vi "Format JSON.vi"(8 "error in (no error)":errorcluster, 11 "String":string) -> (0 "error out":errorcluster, 3 "String out":string)   [LabVIEW 2015, in "Project.lvclass"]
uses:
  Project.lvclass
panel:
  # "Test:5"
  # "\"Test:5,Test1:6\""
  # "\"{\"\"Test\"\":5,\"\"Test1\"\":6}\""
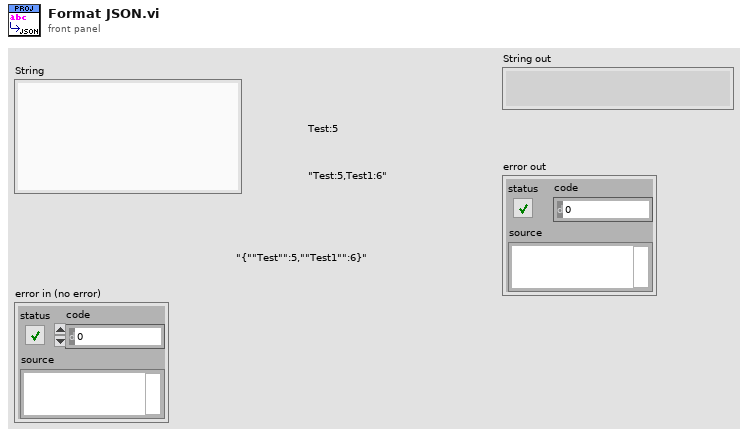
[diagram p1: front panel]
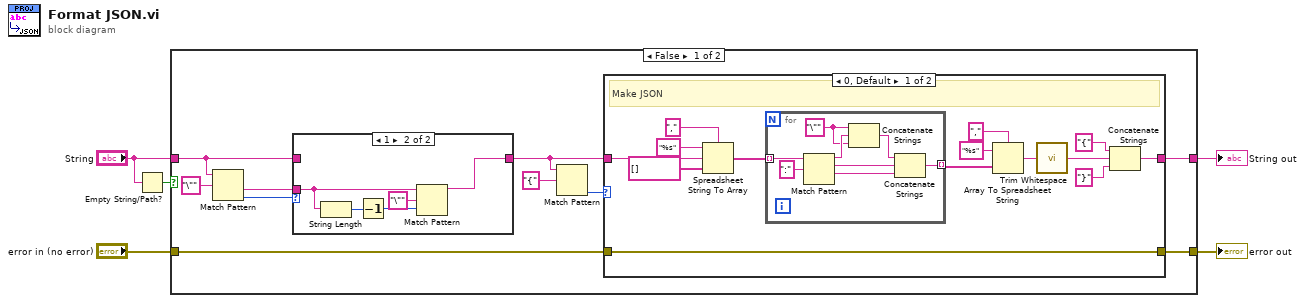
[diagram p0: block diagram]
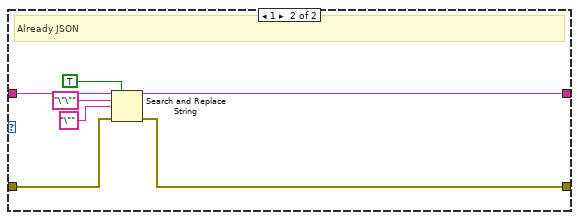
[diagram p2: hidden frame]
diagram:
  n1 = Empty String/Path?(string/path="String") -> (empty?=w5:bool)
  n2 = case shown="False" w5 {
    tunnel: "String" -> [w12 w52]
    tunnel: [w11 w52] -> w1
    tunnel: "error in (no error)" -> [w10 w51]
    tunnel: [w9 w51] -> w2
    frame False {
      n3 = Match Pattern(string=w12, regular expression="\"") -> (after substring=w14:string, offset past match=w13:i32)  [unwired: 1 in, 2 out]
      n4 = case shown="1" w13 {
        tunnel: w14 -> [_ w48]
        tunnel: [w45 w49] -> w7
        tunnel: w12 -> [w45 _]
        frame -1, Default {
        }
        frame 1 {
          n5 = String Length(string=w48) -> (length=w47:i32)
          n6 = Decrement(x=w47) -> (x-1=w46:i32)
          n7 = Match Pattern(string=w48, regular expression="\"", offset (0)=w46) -> (before substring=w49:string)  [unwired: 3 out]
        }
      }
      n8 = Match Pattern(string=w7, regular expression="{") -> (offset past match=w6:i32)  [unwired: 1 in, 3 out]
      n9 = case shown="0, Default" w6 {
        tunnel: [w17 w41] -> w11
        tunnel: w10 -> [w29 w40]
        tunnel: [w29 w39] -> w9
        tunnel: w7 -> [w18 w38]
        frame 0, Default {
          # "Make JSON"
          n10 = Spreadsheet String To Array(delimiter (Tab)=",", format string="%s", spreadsheet string=w18, array type (2D Dbl)=string[] []) -> (array=w25:string[])
          n11 = for {
            tunnel: w25 -> [w37] mode=indexing
            tunnel: [w30] -> w24 mode=indexing
            w31 = "\"" ("string")
            n12 = Match Pattern(string=w37, regular expression=":") -> (before substring=w32:string, match substring=w35:string, after substring=w34:string)  [unwired: 1 in, 1 out]
            n13 = Concatenate Strings(w31, w32, w31) -> (w33:string)
            n14 = Concatenate Strings(w33, w35, w34) -> (w30:string)
          }
          n15 = Array To Spreadsheet String(delimiter (Tab)=",", array=w24, 3:"%s" ("format string")) -> (spreadsheet string=w21:string)
          n16 = call <vilib>:"Trim Whitespace.vi"("string"=w21) -> ("trimmed string"=w16:string)  [unwired: 1 in]
          n17 = Concatenate Strings("{" ("string"), w16, "}" ("string")) -> (w17:string)
        }
        frame 1 {
          # "Already JSON"
          n18 = Search and Replace String(replace all?=TRUE ("replace all? (F)"), input string=w38, search string="\"\"", replace string="\"" ("replace string (\"\")"), error in=w40) -> (result string=w41:string, error out=w39:errorcluster)  [unwired: 3 in, 2 out]
        }
      }
    }
    frame True {
    }
  }
  "error out" <- w2
  "String out" <- w1
